vi "ROS send.vi"(8 "CON IN":T1, 10 "Data in":T2) -> (0 "CON out":T1, 2 "JSON string":string)   [LabVIEW 2015]
uses:
  Control  rossss.ctl
  <vilib>/Intelligent Energy/WebSockets API/WebSockets/WebSockets.lvlib
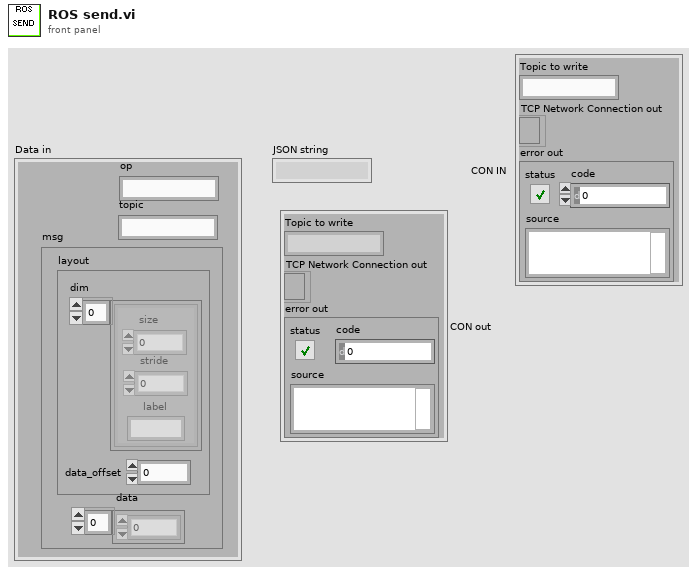
[diagram p1: front panel]
types:
  T1 = cluster{"Topic to write":string, "TCP Network Connection out":refnum<k5>, "error out":errorcluster}
  T2 = typedef "Control  rossss.ctl" = cluster{"op":string, "topic":string, "msg":cluster{"layout":cluster{"dim":cluster{"stride":i16, "size":i16, "label":string}[], "data_offset":dbl}, "data":i32[]}}
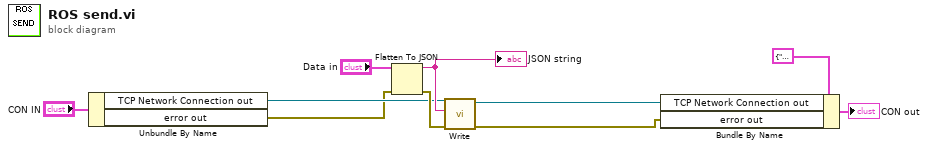
[diagram p0: block diagram]
diagram:
  n1 = Unbundle By Name("CON IN") -> ("TCP Network Connection out"=w6:refnum<k5>, "error out"=w5:errorcluster)
  n2 = Flatten To JSON(anything="Data in", error in (no error)=w5) -> (JSON string=w8:string, 11:w10:errorcluster)  [unwired: 1 in]
  "JSON string" <- w8
  n3 = call <vilib>:"Write.vi"("error in (no error)"=w10, "Data"=w8, "WebSocket Connection in"=w6) -> ("error out"=w2:errorcluster, "WebSocket Connection out"=w3:refnum<k5>)  [unwired: 7 in]
  n4 = Bundle By Name(cluster=T1 {"Topic to write"="", "TCP Network Connection out"=refnum, "error out"={"status"=FALSE, "code"=0, "source"=""}} ("output cluster 2"), "TCP Network Connection out"=w3, "error out"=w2) -> (→"CON out":T1)
